vi "VII Set User Key.vi"(9 "pUserKey":u8[](array[numeric])=[0, 0, 0, 0, 0, 0, 0, 0, 0, 0, 0, 0, 0, 0, 0, 0], 10 "DevIndex":i32, 11 "DevType":i32) -> (3 "function return":i32)   [LabVIEW 2010, in "ControlI2C.lvlib"]
doc: "int __stdcall VII_SetUserKey(int DevType,int DevIndex,unsigned char* pUserKey);"
uses:
  ControlI2C.lvlib
  ControlI2C/Ginkgo_Driver.dll
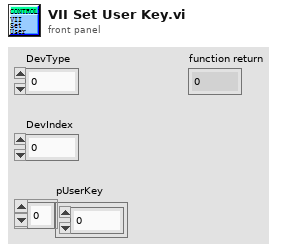
[diagram p1: front panel]
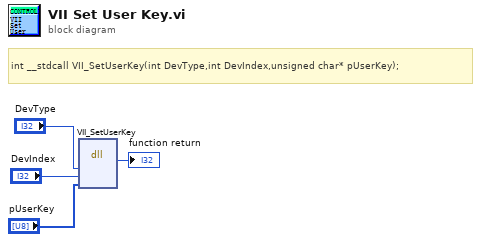
[diagram p0: block diagram]
diagram:
  # "int __stdcall VII_SetUserKey(int DevType,int DevIndex,unsigned char* pUserKey);"
  n1 = dll-call lib="E:/Project/vt_ginkgo/truck/Ginkgo Driver/vs2010/Ginkgo_USB-I2C&SPI&CAN_API_v2.0.3.3/lib/labview_32bit/ControlI2C/Ginkgo_Driver.*" fn="VII_SetUserKey"("DevType"="DevType", "DevIndex"="DevIndex", "pUserKey"="pUserKey") -> (→"function return":i32)  [unwired: 6 in, 2 out]
